vi "Test View.vi"(10 "User Events in":refnum<class "User Events.lvclass">) -> ()   [LabVIEW 2016, in "HPMT_Views.lvlib"]
uses:
  HPMT_Views.lvlib
  User Events/User Events.lvclass
  Typedefs/TestStatus.ctl
  Commands/Command Factory/Command Factory.lvclass
  User Events/User Events.lvclass/User Events.ctl
  Typedefs/StateTypes.ctl
  Commands/Complete Testing Command/Complete Testing Command.lvclass
  Commands/Test One Test Command/Test One Test Command.lvclass
  Typedefs/HPMT_Typedefs.lvlib
panel:
  out "Test One Status":T1
  in  "Test One":bool
  in  "CompleteTest":bool
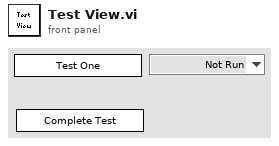
[diagram p1: front panel]
types:
  T1 = typedef "HPMT_Typedefs.lvlib/TestStatus.ctl" = enum16{"Not Run", "Running", "Passed", "Failed"}
  T2 = typedef "HPMT_Typedefs.lvlib/Publish Data Events.ctl" = cluster{"State":refnum<user-event>, "ErrorCode":refnum<user-event>, "Scan Progress":refnum<user-event>, "All Test Status":refnum<user-event>}
  T3 = typedef "HPMT_Typedefs.lvlib/Subscribe Data Events.ctl" = cluster{"Command":refnum<user-event>}
  T4 = cluster{"Event Registration Refnum":refnum<event-registration>}
  T5 = typedef "HPMT_Typedefs.lvlib/StateTypes.ctl" = enum16{"Offline State", "Fault State", "Standby State", "Disabled State", "Enabled State", "Wait For User Input State", "Test Actuator State"}
  T6 = enum8{"Enabled", "Disabled", "Disabled and Grayed Out"}
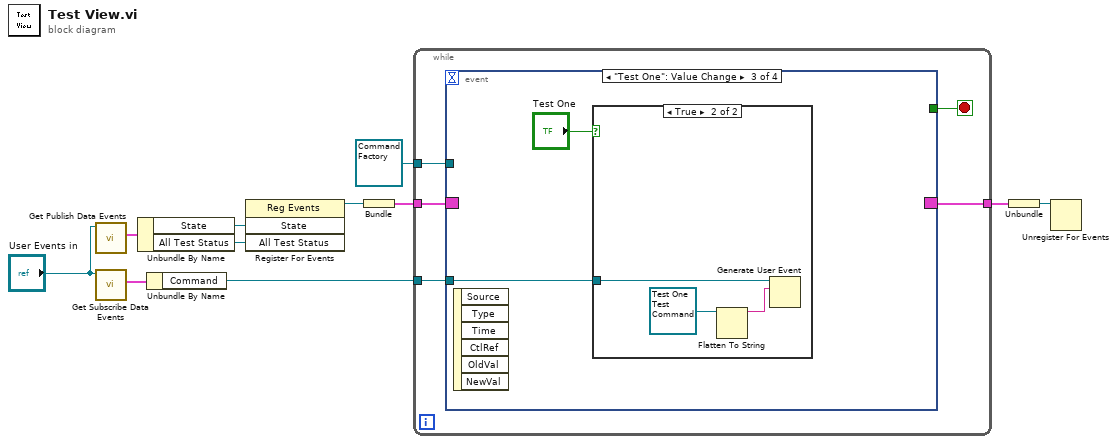
[diagram p0: block diagram]
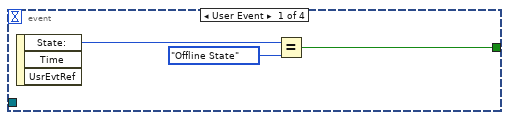
[diagram p2: hidden frame]
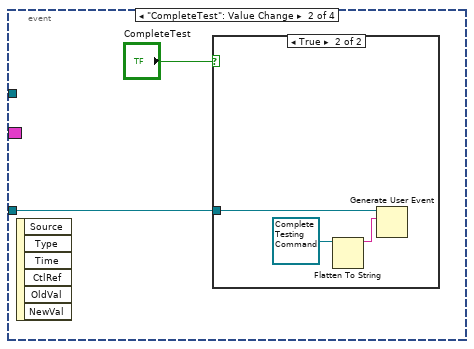
[diagram p3: hidden frame]
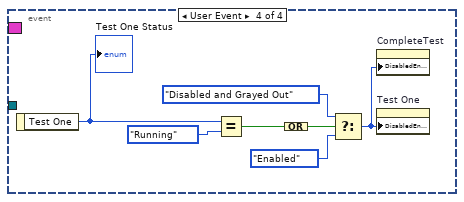
[diagram p6: hidden frame]
diagram:
  n1 = call "Get Publish Data Events.vi"("UserEvents in"="User Events in") -> ("Publish Data Events"=w11:T2)  [unwired: 9 in, 1 out]
  n2 = call "Get Subscribe Data Events.vi"("UserEvents in"="User Events in") -> ("Subscribe Data Events"=w5:T3)  [unwired: 9 in, 1 out]
  n3 = Unbundle By Name(w11) -> ("State"=w10:refnum<user-event>, "All Test Status"=w1:refnum<user-event>)
  n4 = Unbundle By Name(w5) -> ("Command"=w3:refnum<user-event>)
  n5 = register-events(w10, w1) -> (reference out=w9:refnum<event-registration>)  [unwired: 2 in, 1 out]
  n6 = Bundle("Event Registration Refnum"=w9) -> (w6:T4)  [unwired: 1 in]
  n7 = while {
    tunnel: w6 -> [w16]
    tunnel: [w15] -> w7
    tunnel: w3 -> [w13]
    tunnel: refnum<class "Command Factory.lvclass"> refnum ("CommandFactory.lvclass") -> [w12]
    stop <- w14 stop-if-true
    n8 = event shown="[2] \"Test One\": Value Change" {
      selector: w16 -> [_ _ _ _]
      dyn-events: [_ _ _ _] -> w15
      timeout: _ -> [_ _ _ _]
      tunnel: [w18 _ _ _] -> w14
      tunnel: w13 -> [_ w20 w26 _]
      tunnel: w12 -> [_ _ _ _]
      event User Event {
        n9 = event-data() -> ("State:"=w17:T5)  [unwired: 1 in, 2 out]
        n10 = Equal?(x=w17, y=StateTypes."Offline State") -> (x = y?=w18:bool)
      }
      event "CompleteTest": Value Change {
        n11 = event-data() -> ()  [unwired: 1 in, 6 out]
        n12 = case shown="True" "CompleteTest" {
          tunnel: w20 -> [_ w23]
          frame False {
          }
          frame True {
            n13 = Flatten To String(anything=refnum<class "Complete Testing Command.lvclass"> refnum ("Complete Testing Command.lvclass")) -> (data string=w24:string)  [unwired: 3 in, 2 out]
            n14 = Generate User Event(user event=w23, event data cluster=w24) -> ()  [unwired: 2 in, 2 out]
          }
        }
      }
      event "Test One": Value Change {
        n15 = event-data() -> ()  [unwired: 1 in, 6 out]
        n16 = case shown="True" "Test One" {
          tunnel: w26 -> [_ w28]
          frame False {
          }
          frame True {
            n17 = Flatten To String(anything=refnum<class "Test One Test Command.lvclass"> refnum ("Test One Test Command.lvclass")) -> (data string=w29:string)  [unwired: 3 in, 2 out]
            n18 = Generate User Event(user event=w28, event data cluster=w29) -> ()  [unwired: 2 in, 2 out]
          }
        }
      }
      event User Event {
        n19 = event-data() -> ("Test One"=w30:T1)  [unwired: 1 in]
        "Test One Status" <- w30
        n20 = Equal?(x=w30, y=TestStatus."Running") -> (x = y?=w36:bool)
        n21 = Compound Arithmetic op=OR(w36) -> (w35:bool)
        n22 = Select(t=T6."Disabled and Grayed Out", s=w35, f=T6."Enabled" ("Disabled")) -> (s? t:f=w32:T6)
        n23 = property on="CompleteTest" class="Bool"("DisabledEnum"=w32) -> ()  [unwired: 2 in, 2 out]
        n24 = property on="Test One" class="Bool"("DisabledEnum"=w32) -> ()  [unwired: 2 in, 2 out]
      }
    }
  }
  n25 = Unbundle(w7) -> ("Event Registration Refnum"=w8:refnum<event-registration>)
  n26 = Unregister For Events(event registration refnum=w8) -> ()  [unwired: 1 in, 1 out]
